vi "Get_all_data.vi"(8 "error in":errorcluster) -> (0 "error out":errorcluster, 3 "Channel & data arrays out":T1)   [LabVIEW 2017, in "labview-standard-library.lvlib"]
uses:
  labview-standard-library.lvlib
  Channel&data_arrays.ctl
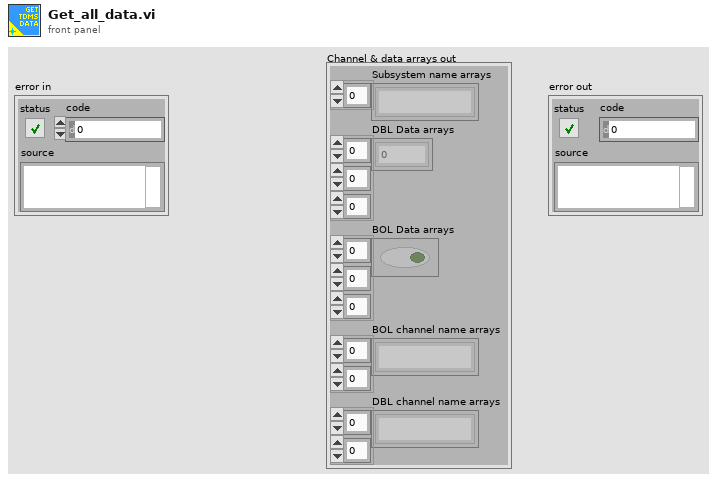
[diagram p1: front panel]
types:
  T1 = typedef "labview-standard-library.lvlib/Channel&data_arrays.ctl" = cluster{"Subsystem name arrays":string[], "DBL Data arrays":dbl[][][], "BOL Data arrays":bool[][][], "BOL channel name arrays":string[][], "DBL channel name arrays":string[][]}
  T2 = typedef "labview-standard-library.lvlib/Subsystem_data.ctl" = cluster{"Subsystem name":string, "Double data points":dbl[][], "Boolean data points":bool[][], "Boolean channel names":string[], "Double channel names":string[]}
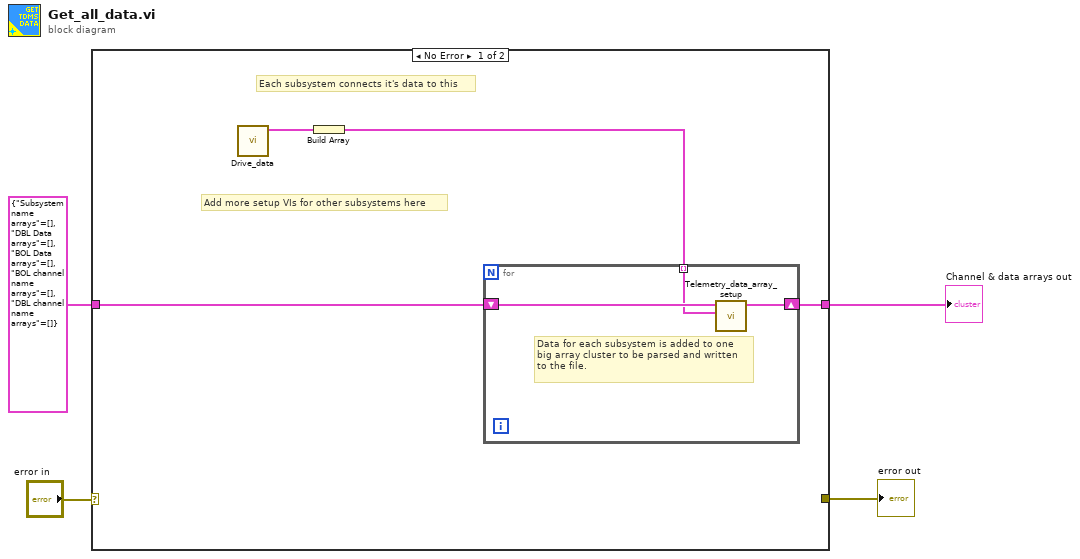
[diagram p0: block diagram]
diagram:
  n1 = case shown="No Error" "error in" {
    selector: "error in" -> [_ w13]
    tunnel: [_ w13] -> w3
    tunnel: [w6 w12] -> w2
    tunnel: T1 {"Subsystem name arrays"=[], "DBL Data arrays"=[], "BOL Data arrays"=[], "BOL channel name arrays"=[], "DBL channel name arrays"=[]} ("Channel & data arrays in") -> [w5 w12]
    frame No Error {
      # "Each subsystem connects it's data to this"
      # "Add more setup VIs for other subsystems here"
      n2 = call "Drive_data.vi"() -> ("Subsystem data out"=w8:T2)  [unwired: 11 in]
      n3 = Build Array(w8) -> (w7:T2[])
      n4 = for {
        tunnel: w7 -> [w10] mode=indexing
        shift-right: [w9] -> w6
        shift-left: w5 -> [w11]
        # "Data for each subsystem is added to one\nbig array cluster to be parsed and written\nto the file."
        n5 = call "Telemetry_data_array_setup.vi"("Subsystem data"=w10, "Channel & data arrays in"=w11) -> ("Channel & data arrays out"=w9:T1)  [unwired: 8 in, 1 out]
      }
    }
    frame Error {
    }
  }
  "error out" <- w3
  "Channel & data arrays out" <- w2
